vi "MechDriveSim_example.vi"() -> ()   [LabVIEW 2019]
uses:
  <vilib>/Rock Robotics/WPI/ThirdParty/JAS_Junk/TrajLib/TypeDef/DIFF_DRIVE_TRAIN_SIM.ctl
  <vilib>/Rock Robotics/WPI/ThirdParty/JAS_Junk/TrajLib/TypeDef/LINEAR_SYSTEM.ctl
  <vilib>/Analysis/Matrix/Datatypes/RealMatrix.ctl
  <vilib>/Rock Robotics/WPI/ThirdParty/JAS_Junk/TrajLib/TypeDef/DCMOTOR.CTL
  <vilib>/Rock Robotics/WPI/ThirdParty/JAS_Junk/TrajLib/Enum/DCMOTOR_TYPES_ENUM.ctl
  <vilib>/Rock Robotics/WPI/ThirdParty/JAS_Junk/TrajLib/Enum/DIFF_DRIVE_ToughBoxMini_GearChoice_ENUM.ctl
  <vilib>/Rock Robotics/WPI/ThirdParty/JAS_Junk/TrajLib/Enum/DIFF_DRIVE_TRAIN_SIM_STATE_ENUM.ctl
  <vilib>/Rock Robotics/WPI/ThirdParty/JAS_Junk/TrajLib/Enum/DIFF_DRIVE_KitBot_WheelSize_ENUM.ctl
  <vilib>/Rock Robotics/WPI/ThirdParty/JAS_Junk/TrajLib/BatterySim_CalculateLoadedBatteryVoltage.vi
  <vilib>/Rock Robotics/WPI/ThirdParty/JAS_Junk/TrajLib/Trajectory_Library.lvlib
  <vilib>/Analysis/Matrix/NI_Matrix.lvlib
panel:
  in  "Tab Control":enum32{"Control", "Simulation"}(tab)
  in  "Motor Dmd - SP\n( +/- 1 )":dbl(slide) scale=-1.0..1.0
  out "Left Motor Vel - PV (Ft/Sec)":dbl format="%20.3f"
  out "Right Motor Vel - PV (Ft/Sec)":dbl format="%20.3f"
  out "Battery Voltage (Volts)":dbl format="%20.3f"
  out "Voltage, Current Chart":cluster{dbl, dbl, "Voltage":dbl}(graph)
  out "PV, SP Chart":T1(graph)
  out "Motor Current  - Left (Amps)":dbl format="%20.3f"
  out "Motor Current  - Right (Amps)":dbl format="%20.3f"
  out "Right Motor Dist (Ft)":dbl format="%20.3f"
  out "Left Motor Dist (Ft)":dbl format="%20.3f"
  out "Gyro Heading (Deg)":dbl format="%20.3f"
  out "Differential Drive Train Sim":T2 {"m_Motor"."Jr_KgM2" format="%13.5p"; "m_Motor"."L_H" format="%13.5p"; "m_Motor"."Kt_NMPerAmp" format="%13.5p"; "m_Motor"."KvINV_RadPerSecPerVolt" format="%13.5p"; "m_Motor"."R_Ohms" format="%13.5p"; "m_Motor"."FreeSpeed_RadPerSec" format="%13.5p"; "m_Motor"."FreeCurrent_Amps" format="%13.5p"; "m_Motor"."StallCurrent_Amps" format="%13.5p"; "m_Motor"."StallTorque_NM" format="%13.5p"; "m_Motor"."nominalVoltage_Volts" format="%13.5p"}
  # "<States, 1>"
  # "<Outputs, 1>"
  # "<Inputs, 1>"
  # "<Outputs, 1>"
  # "<States,States>"
  # "<States,Inputs>"
  # "<Outputs,States>"
  # "<Outputs,Inputs>"
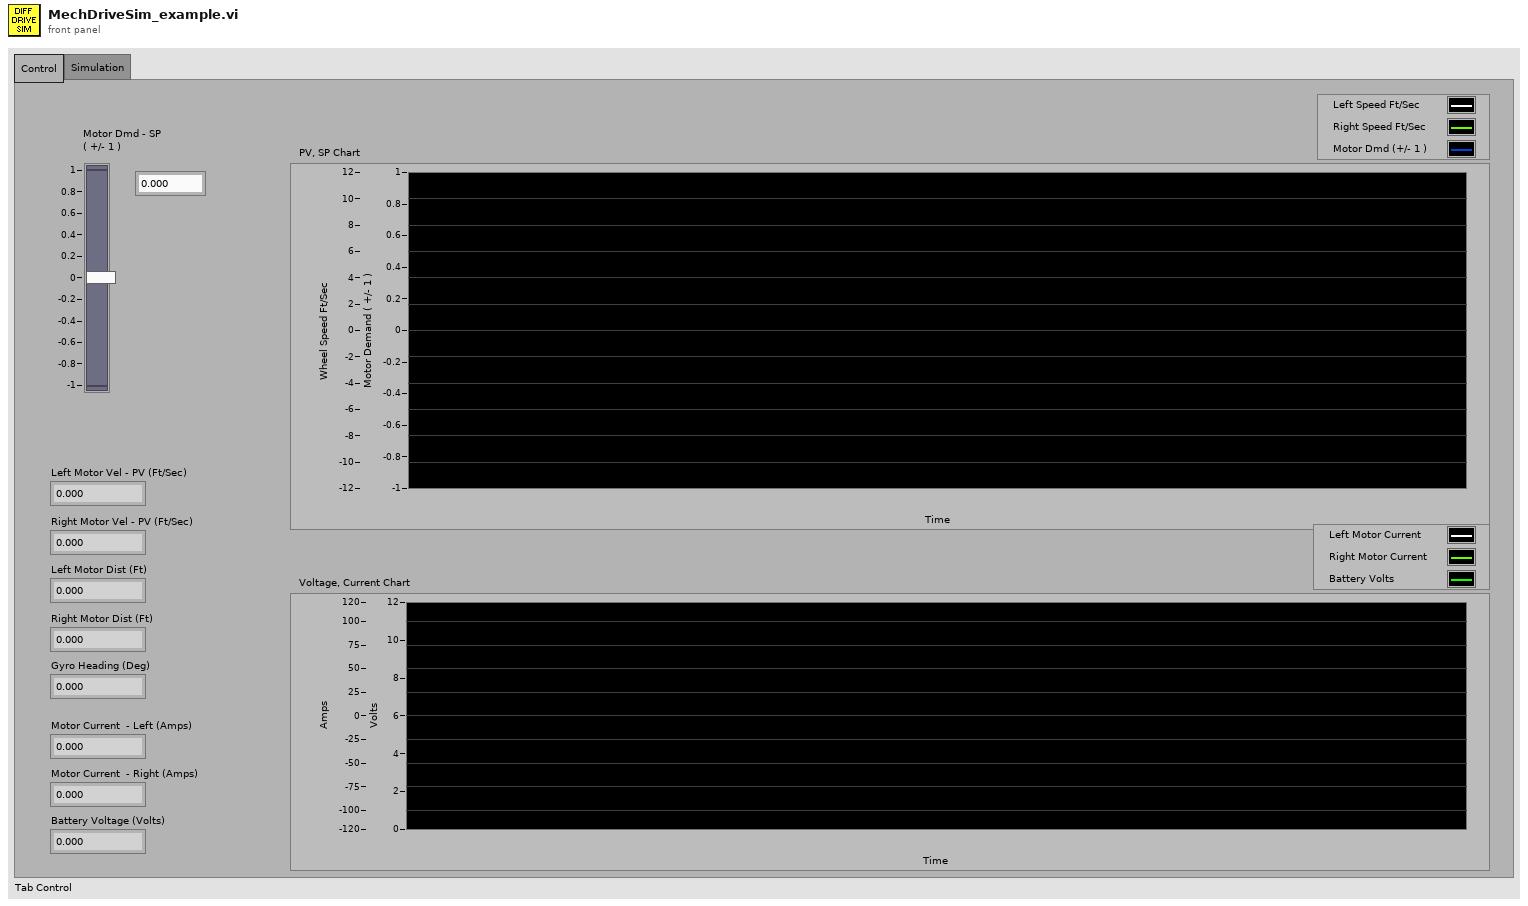
[diagram p1: front panel]
types:
  T1 = cluster{"upper limit":dbl, "Real Matrix Element":dbl, "Real Matrix Element":dbl}
  T2 = typedef "Trajectory_Library.lvlib/DIFF_DRIVE_TRAIN_SIM.ctl" = cluster{"m_Plant":T3, "m_X":T4, "m_Y":T4, "m_U":T4, "MeasureStdDev":T4, "m_Motor":T5, "m_OriginalGearing":dbl, "m_CurrentGearing":dbl, "m_WheelRadius_M":dbl, "m_RB":dbl}
  T3 = typedef "Trajectory_Library.lvlib/LINEAR_SYSTEM.ctl" = cluster{"m_A":T4, "m_B":T4, "m_C":T4, "m_D":T4, "States":i32, "Inputs":i32, "Outputs":i32}
  T4 = typedef "NI_Matrix.lvlib/RealMatrix.ctl" = dbl[][]
  T5 = typedef "Trajectory_Library.lvlib/DCMOTOR.CTL" = cluster{"nominalVoltage_Volts":dbl, "StallTorque_NM":dbl, "StallCurrent_Amps":dbl, "FreeCurrent_Amps":dbl, "FreeSpeed_RadPerSec":dbl, "R_Ohms":dbl, "KvINV_RadPerSecPerVolt":dbl, "Kt_NMPerAmp":dbl, "L_H":dbl, "Jr_KgM2":dbl}
  T6 = typedef "Trajectory_Library.lvlib/DIFF_DRIVE_TRAIN_SIM_STATE_ENUM.ctl" = enum16{"X_POS", "Y_POS", "HEADING", "LEFT_VEL", "RIGHT_VEL", "LEFT_DIST", "RIGHT_DIST"}
  T7 = typedef "Trajectory_Library.lvlib/DIFF_DRIVE_KitBot_WheelSize_ENUM.ctl" = enum16{"4 Inch", "6 Inch", "8 Inch", "10 Inch"}
  T8 = typedef "Trajectory_Library.lvlib/DIFF_DRIVE_ToughBoxMini_GearChoice_ENUM.ctl" = enum16{"Ratio_12_75", "Ratio_10_71", "Ratio_8_45", "Ratio_7_31", "Ratio_5_95"}
  T9 = typedef "Trajectory_Library.lvlib/DCMOTOR_TYPES_ENUM.ctl" = enum16{"CIM", "AndyMark 9015", "Andy Mark RS 775 125", "Bag", "BaneBots RS 550", "BaneBots RS 775", "Falcon 500", "Mini CIM", "NEO", "NEO 550", "Romi BuiltIn", "Vex 775 Pro", "Snow Blower AM 2235A", "Bosch Seat AM 3493"}
  T10 = cluster{"Feet":dbl, "Feet":dbl, "Motor Dmd - SP\n( +/- 1 )":dbl}
  T11 = typedef "Trajectory_Library.lvlib/DIFF_DRIVE_SIM_SIMULATION_PARAMS.ctl" = cluster{"X Pos Meas Std Dev M":dbl, "Y Pos Meas Std Dev M":dbl, "Heading Meas Std Dev Rad":dbl, "Left Vel Meas Std Dev M/S":dbl, "Right Vel Meas Std Dev M/S":dbl, "Left Pos Meas Std Dev M":dbl, "Right Pos Meas Std Dev M":dbl}
  T12 = typedef "Trajectory_Library.lvlib/DIFF_DRIVE_SIM_MODEL_PARAMS.CTL" = cluster{"TracWidth_M":dbl, "WheelRadius_M":dbl, "Gearing":dbl, "Mass kg":dbl, "MOI kgm2":dbl, "DCMOTOR_TYPES":T9, "Num Motors":i32}
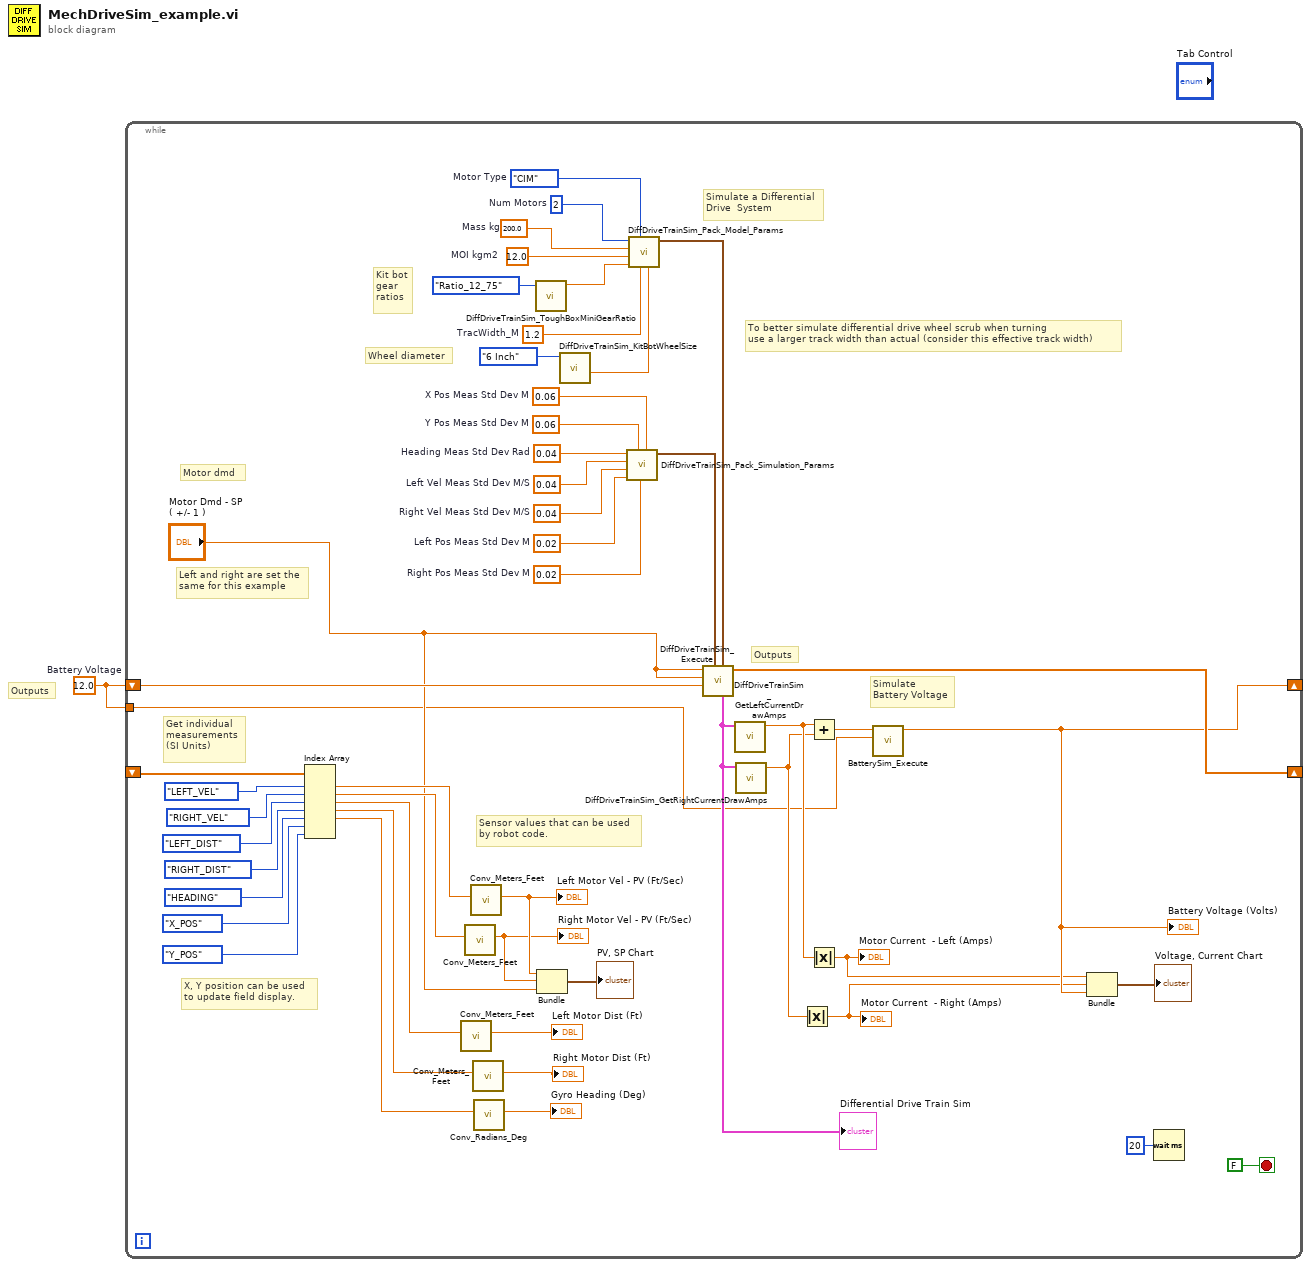
[diagram p0: block diagram]
diagram:
  w1 = 12.0  # Battery Voltage
  # "Outputs"
  n1 = while {
    shift-right: [w23] -> _
    shift-left: w1 -> [w24]
    shift-right: [w48] -> _
    shift-left: _ -> [w32]
    tunnel: w1 -> [w4]
    stop <- FALSE stop-if-true
    w36 = 200.0  # Mass kg
    w37 = 12.0  # MOI kgm2
    w38 = 1.2  # TracWidth_M
    w39 = 0.04  # Heading Meas Std Dev Rad
    w40 = 0.04  # Left Vel Meas Std Dev M/S
    w41 = 0.04  # Right Vel Meas Std Dev M/S
    w42 = 0.02  # Left Pos Meas Std Dev M
    w43 = 0.06  # Y Pos Meas Std Dev M
    w44 = 0.02  # Right Pos Meas Std Dev M
    w45 = 0.06  # X Pos Meas Std Dev M
    w51 = 2  # Num Motors
    w52 = DCMOTOR_TYPES_ENUM."CIM"  # Motor Type
    # "To better simulate differential drive wheel scrub when turning\nuse a larger track width than actual (consider this effective track width)"
    # "Sensor values that can be used\nby robot code."
    # "X, Y position can be used\nto update field display."
    # "Left and right are set the\nsame for this example"
    # "Motor dmd"
    # "Wheel diameter"
    # "Get individual\nmeasurements\n(SI Units)"
    # "Kit bot\ngear \nratios"
    # "Outputs"
    # "Simulate\nBattery Voltage"
    # "Simulate a Differential\nDrive  System"
    n2 = Index Array(array=w32, index #1=DIFF_DRIVE_TRAIN_SIM_STATE_ENUM."LEFT_VEL" ("DIFF_DRIVE_TRAIN_SIM_STATE"), index #2=DIFF_DRIVE_TRAIN_SIM_STATE_ENUM."RIGHT_VEL" ("DIFF_DRIVE_TRAIN_SIM_STATE"), index #3=DIFF_DRIVE_TRAIN_SIM_STATE_ENUM."LEFT_DIST" ("DIFF_DRIVE_TRAIN_SIM_STATE"), index #4=DIFF_DRIVE_TRAIN_SIM_STATE_ENUM."RIGHT_DIST" ("DIFF_DRIVE_TRAIN_SIM_STATE"), index #5=DIFF_DRIVE_TRAIN_SIM_STATE_ENUM."HEADING" ("DIFF_DRIVE_TRAIN_SIM_STATE"), index #6=DIFF_DRIVE_TRAIN_SIM_STATE_ENUM."X_POS" ("DIFF_DRIVE_TRAIN_SIM_STATE"), index #7=DIFF_DRIVE_TRAIN_SIM_STATE_ENUM."Y_POS" ("DIFF_DRIVE_TRAIN_SIM_STATE")) -> (element #1=w21:dbl, element #2=w20:dbl, element #3=w15:dbl, element #4=w14:dbl, element #5=w5:dbl)  [unwired: 2 out]
    n3 = call <vilib>:"Conv_Meters_Feet.vi"("Meters"=w15) -> ("Feet"=→"Left Motor Dist (Ft)":dbl)  [unwired: 10 in]
    n4 = call <vilib>:"Conv_Meters_Feet.vi"("Meters"=w20) -> ("Feet"=w18:dbl)  [unwired: 10 in]
    "Right Motor Vel - PV (Ft/Sec)" <- w18
    n5 = call <vilib>:"Conv_Meters_Feet.vi"("Meters"=w21) -> ("Feet"=w19:dbl)  [unwired: 10 in]
    "Left Motor Vel - PV (Ft/Sec)" <- w19
    n6 = call <vilib>:"Conv_Meters_Feet.vi"("Meters"=w14) -> ("Feet"=→"Right Motor Dist (Ft)":dbl)  [unwired: 10 in]
    n7 = call <vilib>:"Conv_Radians_Deg.vi"("Radians"=w5) -> ("Degrees"=→"Gyro Heading (Deg)":dbl)  [unwired: 10 in]
    n8 = call <vilib>:"DiffDriveTrainSim_ToughBoxMiniGearRatio.vi"("ToughBoxMiniGear"=DIFF_DRIVE_ToughBoxMini_GearChoice_ENUM."Ratio_12_75") -> ("GearRatio"=w34:dbl)  [unwired: 10 in]
    n9 = Bundle("Feet"=w19, "Feet"=w18, "Motor Dmd - SP\n( +/- 1 )"="Motor Dmd - SP\n( +/- 1 )") -> (→"PV, SP Chart":T10)  [unwired: 1 in]
    n10 = call <vilib>:"DiffDriveTrainSim_KitBotWheelSize.vi"("Wheel Size"=DIFF_DRIVE_KitBot_WheelSize_ENUM."6 Inch") -> ("WheelRadius_M"=w25:dbl)  [unwired: 9 in, 1 out]
    n11 = call <vilib>:"DiffDriveTrainSim_Pack_Simulation_Params.vi"("X Pos Meas Std Dev M"=w45, "Right Pos Meas Std Dev M"=w44, "Y Pos Meas Std Dev M"=w43, "Left Pos Meas Std Dev M"=w42, "Right Vel Meas Std Dev M/S"=w41, "Left Vel Meas Std Dev M/S"=w40, "Heading Meas Std Dev Rad"=w39) -> ("DiffDriveSim_Simulation _Params"=w46:T11)  [unwired: 4 in]
    n12 = call <vilib>:"DiffDriveTrainSim_Pack_Model_Params.vi"("WheelRadius_M"=w25, "TracWidth_M"=w38, "DCMOTOR_TYPES"=w52, "Gearing"=w34, "MOI kgm2"=w37, "Mass kg"=w36, "Num Motors"=w51) -> ("DiffDriveSim_Model _Params"=w47:T12)  [unwired: 4 in]
    n13 = call <vilib>:"DiffDriveTrainSim_Execute.vi"("LinearSystem_ID_DiffDrv_Model"=w47, "DiffDriveSim_Simulation _Params"=w46, "BatteryVoltage"=w24, "Right Motor Dmd"="Motor Dmd - SP\n( +/- 1 )", "Left Motor Dmd"="Motor Dmd - SP\n( +/- 1 )") -> ("Outputs"=w48:dbl[], "out DiffDriveTrainSim"=w22:T2)  [unwired: 4 in, 1 out]
    "Differential Drive Train Sim" <- w22
    n14 = call <vilib>:"DiffDriveTrainSim_GetLeftCurrentDrawAmps.vi"("DiffDriveTrainSim"=w22) -> ("LeftCurrentDraw_Amps"=w10:dbl)  [unwired: 10 in]
    n15 = call <vilib>:"DiffDriveTrainSim_GetRightCurrentDrawAmps.vi"("DiffDriveTrainSim"=w22) -> ("RightCurrentDraw_Amps"=w9:dbl)  [unwired: 10 in]
    n16 = Absolute Value(x=w9) -> (abs(x)=w7:dbl)
    "Motor Current  - Right (Amps)" <- w7
    n17 = Add(x=w10, y=w9) -> (x+y=w33:dbl)
    n18 = Absolute Value(x=w10) -> (abs(x)=w8:dbl)
    "Motor Current  - Left (Amps)" <- w8
    n19 = call <vilib>:"BatterySim_Execute.vi"("Nominal Battery Voltage"=w4, "Current"=w33) -> ("Voltage"=w23:dbl)  [unwired: 9 in]
    "Battery Voltage (Volts)" <- w23
    n20 = Bundle(w8, w7, "Voltage"=w23) -> (→"Voltage, Current Chart":cluster{dbl, dbl, "Voltage":dbl})  [unwired: 1 in]
    n21 = Wait (ms)(milliseconds to wait=u32 20) -> ()  [unwired: 1 out]
  }
